vi "Periodic Tasks.vi"(8 "error in":errorcluster) -> ()   [LabVIEW 2018]
doc: "This VI runs in parallel to other robot code. It can contain as many user-defined periodic loops as you need. These can carry out PID or other sorts of timed response."
uses:
  <vilib>/Rock Robotics/WPI/Utilities/WPI_GetSetVariantRefNum.vi
  Robot Global Data.vi
panel:
  out "Cargo Stop Current":dbl=10.0 format="%#_13g"
  out "Stop the grabber":bool
  out "Solenoid Voltage":dbl
  out "Input Voltage":dbl
  out "Compressor current (A)":dbl
  out "all currents (A)":dbl[](array[numeric]) caption="0\n1\n2\n3\n4\n5\n6\n7\n8\n9\n10\n11\n12\n13\n14\n15"
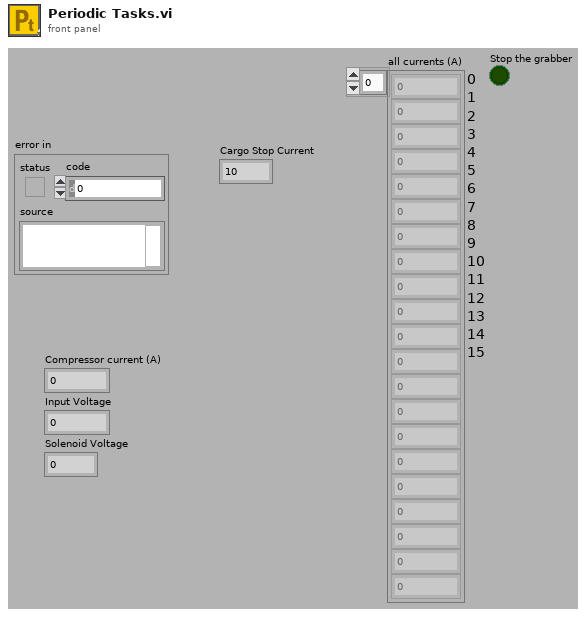
[diagram p1: front panel]
types:
  T1 = typedef "WPI_JoystickDevRef.ctl" = cluster{"Device":T2}
  T2 = typedef "WPI_JoystickDeviceEnum.ctl" = enum16{"USB 0", "USB 1", "USB 2", "USB 3", "USB 4", "USB 5"}
  T3 = cluster{"JoystickDevRef":T1, "JoystickDevRef":T1}
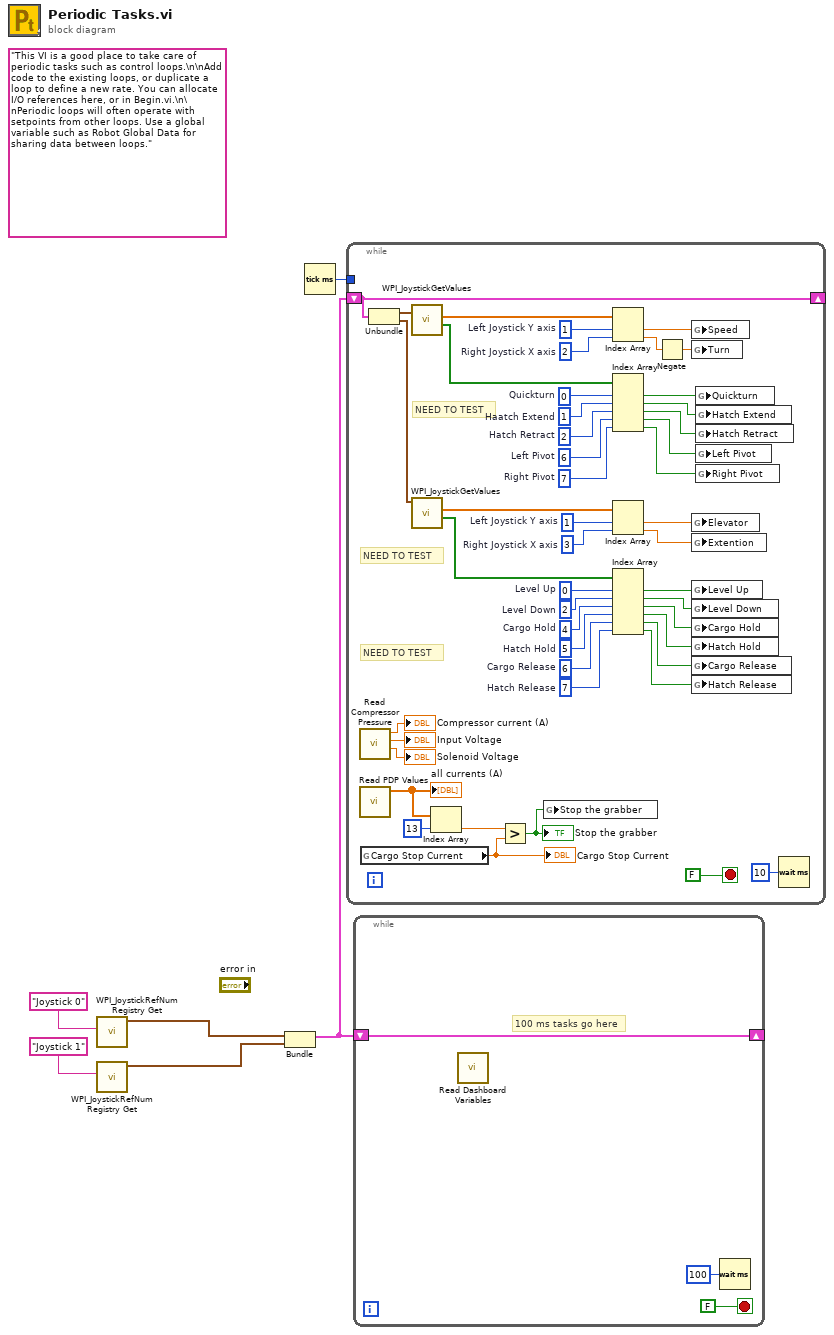
[diagram p0: block diagram]
diagram:
  (unwired) "This VI is a good place to take care of periodic tasks such as control loops.\n\nAdd code to the existing loops, or duplicate a loop to define a new rate. You can allocate I/O references here, or in Begin.vi.\n\nPeriodic loops will often operate with setpoints from other loops. Use a global variable such as Robot Global Data for sharing data between loops."
  n1 = call <vilib>:"WPI_JoystickRefNum Registry Get.vi"("refnum name"="Joystick 0") -> ("JoystickDevRef"=w3:T1)  [unwired: 1 in, 9 out]
  n2 = call <vilib>:"WPI_JoystickRefNum Registry Get.vi"("refnum name"="Joystick 1") -> ("JoystickDevRef"=w1:T1)  [unwired: 1 in, 9 out]
  n3 = Bundle("JoystickDevRef"=w3, "JoystickDevRef"=w1) -> (w2:T3)  [unwired: 1 in]
  n4 = Tick Count (ms)() -> (millisecond timer value=w5:u32)
  n5 = while {
    shift-right: [w48] -> _
    shift-left: w2 -> [w48]
    tunnel: w5 -> [_]
    stop <- FALSE stop-if-true
    w7 = 7  # Right Pivot
    w8 = 6  # Left Pivot
    w17 = 7  # Hatch Release
    w18 = 6  # Cargo Release
    w19 = 5  # Hatch Hold
    w20 = 4  # Cargo Hold
    w21 = 2  # Level Down
    w22 = 0  # Level Up
    w26 = 3  # Right Joystick X axis
    w27 = 1  # Left Joystick Y axis
    w30 = 2  # Hatch Retract
    w31 = 1  # Haatch Extend
    w32 = 0  # Quickturn
    w42 = 2  # Right Joystick X axis
    w43 = 1  # Left Joystick Y axis
    # "NEED TO TEST"
    # "NEED TO TEST"
    # "NEED TO TEST"
    n6 = call "Read Compressor Pressure.vi"() -> ("Solenoid Voltage"=→"Solenoid Voltage":dbl, "Input Voltage"=→"Input Voltage":dbl, "Compressor current (A)"=→"Compressor current (A)":dbl)  [unwired: 9 in]
    n7 = call "Read PDP Values.vi"() -> ("all currents (A)"=w34:dbl[])  [unwired: 11 in]
    "all currents (A)" <- w34
    n8 = global read "Robot Global Data.vi" "Cargo Stop Current"() -> (w23:dbl)
    "Cargo Stop Current" <- w23
    n9 = Unbundle(w48) -> ("JoystickDevRef"=w47:T1, "JoystickDevRef"=w44:T1)
    n10 = call <vilib>:"WPI_JoystickGetValues.vi"("JoystickDevRef"=w47) -> ("Buttons"=w50:bool[], "Axes"=w52:dbl[])  [unwired: 6 in, 3 out]
    n11 = call <vilib>:"WPI_JoystickGetValues.vi"("JoystickDevRef"=w44) -> ("Buttons"=w46:bool[], "Axes"=w45:dbl[])  [unwired: 6 in, 3 out]
    n12 = Index Array(array=w34, index=13) -> (element=w36:dbl)
    n13 = Greater?(x=w36, y=w23) -> (0:w33:bool)
    "Stop the grabber" <- w33
    n14 = global write "Robot Global Data.vi" "Stop the grabber"(w33) -> ()
    n15 = Index Array(array=w52, index #1=w43, index #2=w42) -> (element #1=w41:dbl, element #2=w40:dbl)
    n16 = Index Array(array=w50, index #1=w32, index #2=w31, index #3=w30, index #4=w8, index #5=w7) -> (element #1=w49:bool, element #2=w29:bool, element #3=w28:bool, element #4=w10:bool, element #5=w9:bool)
    n17 = Index Array(array=w45, index #1=w27, index #2=w26) -> (element #1=w25:dbl, element #2=w24:dbl)
    n18 = Index Array(array=w46, index #1=w22, index #2=w21, index #3=w20, index #4=w19, index #5=w18, index #6=w17) -> (element #1=w16:bool, element #2=w15:bool, element #3=w14:bool, element #4=w13:bool, element #5=w12:bool, element #6=w11:bool)
    n19 = Negate(x=w40) -> (-x=w51:dbl)
    n20 = global write "Robot Global Data.vi" "Speed"(w41) -> ()
    n21 = global write "Robot Global Data.vi" "Turn"(w51) -> ()
    n22 = global write "Robot Global Data.vi" "Elevator"(w25) -> ()
    n23 = global write "Robot Global Data.vi" "Extention"(w24) -> ()
    n24 = global write "Robot Global Data.vi" "Level Up"(w16) -> ()
    n25 = global write "Robot Global Data.vi" "Level Down"(w15) -> ()
    n26 = global write "Robot Global Data.vi" "Cargo Hold"(w14) -> ()
    n27 = global write "Robot Global Data.vi" "Hatch Hold"(w13) -> ()
    n28 = global write "Robot Global Data.vi" "Cargo Release"(w12) -> ()
    n29 = global write "Robot Global Data.vi" "Hatch Release"(w11) -> ()
    n30 = global write "Robot Global Data.vi" "Quickturn"(w49) -> ()
    n31 = global write "Robot Global Data.vi" "Hatch Extend"(w29) -> ()
    n32 = global write "Robot Global Data.vi" "Hatch Retract"(w28) -> ()
    n33 = global write "Robot Global Data.vi" "Left Pivot"(w10) -> ()
    n34 = global write "Robot Global Data.vi" "Right Pivot"(w9) -> ()
    n35 = Wait (ms)(milliseconds to wait=u32 10) -> ()  [unwired: 1 out]
  }
  n36 = while {
    shift-right: [w55] -> _
    shift-left: w2 -> [w55]
    stop <- FALSE stop-if-true
    # "100 ms tasks go here"
    n37 = call "Read Dashboard Variables.vi"() -> ()  [unwired: 12 in]
    n38 = Wait (ms)(milliseconds to wait=u32 100) -> ()  [unwired: 1 out]
  }
